vi "Save Configuration File.vi"(8 "Files To Acquire":i32, 10 "Data File I/O Information":T1={"Name of Configuration"="", "Path"=path "C:/Users/Achilles/Data/12-20-00", "File Name"="Whole Gel Image", "Files To Acquire"=1, "Current File Number"=21, "Time Limit"=1.0, "Save Data"=FALSE, "Additional Comments"=""}, 11 "Configuration File Path":path=path "") -> (3 "new file path":path)   [LabVIEW 2009]
uses:
  Acquisition Settings.vi
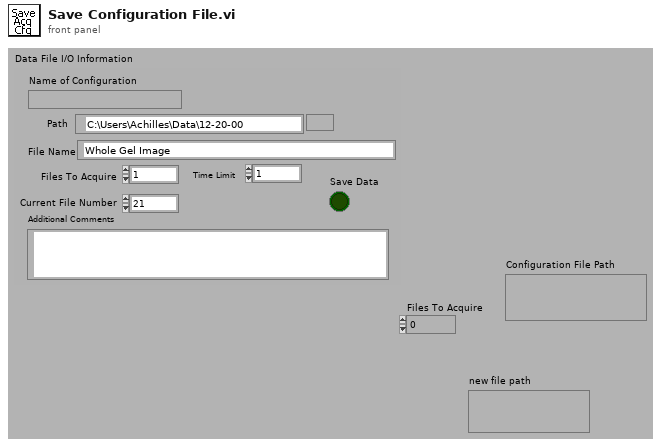
[diagram p1: front panel]
types:
  T1 = cluster{"Name of Configuration":string, "Path":path, "File Name":string, "Files To Acquire":i32, "Current File Number":i32, "Time Limit":dbl, "Save Data":bool, "Additional Comments":string}
  T2 = enum16{"open", "open or create", "create or replace", "create", "open (read only)"}
  T3 = cluster{"Name":string, "Signal Routing":cluster{"signal name":u16, "signal source":u16, "signal source line number":u32, "signal name line number":u32}[]}[]
  T4 = cluster{"Name":string, "Device Number":i16, "Counter Number":i16, "Line Type for Gate":u32, "Line Number for Gate":u32, "Line Type for Source":u32, "Line Number for Source":u32, "Transfer Method":u32, "Signal Routing Configuration":i16}[]
  T5 = cluster{"Device Number":i16, "Counter Number":i16, "Signal Routing Configuration":i16}
  T6 = cluster{"device":i16, "channel":tag, "buffer size":i32, "Signal Description":cluster{"Name":string, "signal type":enum16{"Sine Wave", "Square Wave", "Sawtooth", "Triangle Wave"}, "period":dbl, "amplitude":dbl, "phase (0 deg)":dbl, "offset (0.0)":dbl, "resting voltage":dbl, "% duty cycle":dbl}[], "clock source (internal:1)":u16, "Clock Line Number":i16}[]
  T7 = cluster{"Name":string, "Device Number":i16, "Counter Number":i16, "Pulse Spec 1 (Clocks)":u32, "Pulse Spec 2 (Clocks)":u32, "Signal Routing Configuration":i16, "Inverted":bool}[]
  T8 = cluster{"Device Number":i16, "Counter Number":i16, "Line Type for Source":u32, "Line Number for Source":u32, "Signal Routing Configuration":i16}
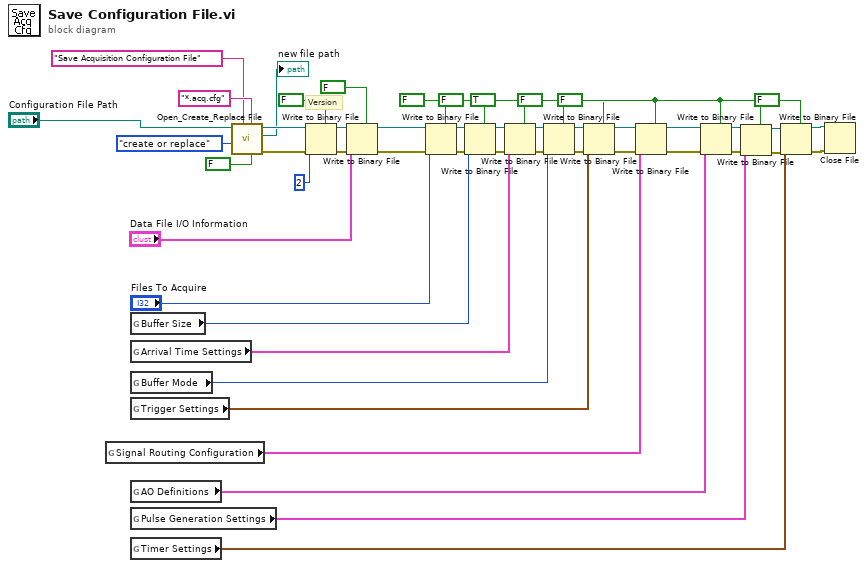
[diagram p0: block diagram]
diagram:
  w9 = TRUE ("header (F)")
  # "Version"
  n1 = global read "Acquisition Settings.vi" "Signal Routing Configuration"() -> (w10:T3)
  n2 = global read "Acquisition Settings.vi" "Buffer Size"() -> (w32:i32)
  n3 = global read "Acquisition Settings.vi" "Arrival Time Settings"() -> (w31:T4)
  n4 = global read "Acquisition Settings.vi" "Buffer Mode"() -> (w30:u32)
  n5 = global read "Acquisition Settings.vi" "Trigger Settings"() -> (w29:T5)
  n6 = global read "Acquisition Settings.vi" "AO Definitions"() -> (w28:T6)
  n7 = global read "Acquisition Settings.vi" "Pulse Generation Settings"() -> (w27:T7)
  n8 = global read "Acquisition Settings.vi" "Timer Settings"() -> (w26:T8)
  n9 = call <vilib>:"Open_Create_Replace File.vi"("advisory dialog? (display:T)"=FALSE, "pattern"="*.acq.cfg", "prompt"="Save Acquisition Configuration File", "function (open:0)"=T2."create or replace", "file path"="Configuration File Path") -> ("error out"=w47:errorcluster, "new file path"=→"new file path":path, "refnum"=w48:refnum<file>)  [unwired: 3 in, 1 out]
  n10 = Write to Binary File(file (use dialog)=w48, data=2, error in=w47, 5:FALSE ("prepend array or string size? (T)")) -> (refnum out=w44:refnum<file>, error out=w39:errorcluster)  [unwired: 2 in, 1 out]
  n11 = Write to Binary File(file (use dialog)=w44, data="Data File I/O Information", error in=w39, 5:FALSE ("prepend array or string size? (T)")) -> (refnum out=w16:refnum<file>, error out=w15:errorcluster)  [unwired: 2 in, 1 out]
  n12 = Write to Binary File(file (use dialog)=w16, data="Files To Acquire", error in=w15, 5:FALSE ("prepend array or string size? (T)")) -> (refnum out=w43:refnum<file>, error out=w38:errorcluster)  [unwired: 2 in, 1 out]
  n13 = Write to Binary File(file (use dialog)=w43, data=w32, error in=w38, 5:FALSE ("prepend array or string size? (T)")) -> (refnum out=w42:refnum<file>, error out=w37:errorcluster)  [unwired: 2 in, 1 out]
  n14 = Write to Binary File(file (use dialog)=w42, data=w31, error in=w37, 5:w9) -> (refnum out=w41:refnum<file>, error out=w36:errorcluster)  [unwired: 2 in, 1 out]
  n15 = Write to Binary File(file (use dialog)=w41, data=w30, error in=w36, 5:FALSE ("prepend array or string size? (T)")) -> (refnum out=w40:refnum<file>, error out=w35:errorcluster)  [unwired: 2 in, 1 out]
  n16 = Write to Binary File(file (use dialog)=w40, data=w29, error in=w35, 5:FALSE ("prepend array or string size? (T)")) -> (refnum out=w14:refnum<file>, error out=w13:errorcluster)  [unwired: 2 in, 1 out]
  n17 = Write to Binary File(file (use dialog)=w14, data=w10, error in=w13, 5:w9) -> (refnum out=w11:refnum<file>, error out=w12:errorcluster)  [unwired: 2 in, 1 out]
  n18 = Write to Binary File(file (use dialog)=w11, data=w28, error in=w12, 5:w9) -> (refnum out=w23:refnum<file>, error out=w22:errorcluster)  [unwired: 2 in, 1 out]
  n19 = Write to Binary File(file (use dialog)=w23, data=w27, error in=w22, 5:w9) -> (refnum out=w20:refnum<file>, error out=w21:errorcluster)  [unwired: 2 in, 1 out]
  n20 = Write to Binary File(file (use dialog)=w20, data=w26, error in=w21, 5:FALSE ("prepend array or string size? (T)")) -> (refnum out=w24:refnum<file>, error out=w25:errorcluster)  [unwired: 2 in, 1 out]
  n21 = Close File(refnum=w24, error in=w25) -> ()  [unwired: 2 out]
